vi "Main.vi"() -> ()   [LabVIEW 2021]
doc: "This vi acts as an user interface to display acquire data and save data when required. User can ineract with the panel to choose file (CSV or TDMS) and data display type(chart or graph). It also allow user to select channel index and define channel name, scale and offset. It then can let user choose a moment to start recording either on defined time length or user choice. Additional functionality of a control loop for the Cryocooler Instron project."
uses:
  Control/Data Display Choice Enum.ctl
  Control/File Choice Enum.ctl
  Control/User Interface Reference Cluster.ctl
  Control/Output Data Cluster.ctl
  Control/Command and Data Cluster.ctl
  Control/Data Display Manager Enum.ctl
  Control/Volt Chl.ctl
  Control/File Manager Enum.ctl
  Control/DAQ Manager Enum.ctl
  <vilib>/Analysis/baseanly.llb/Mean (DBL).vi
  <extravilib>/ChannelInstances/Tag-bool/Write With Abort.vi
  <extravilib>/ChannelInstances/Tag-a[.](wfm(dbl))/Read With Abort.vi
  <extravilib>/ChannelInstances/Tag-bool/Read With Abort.vi
  <extravilib>/ChannelInstances/Stream-a[.](wfm(dbl))/Read With Abort.vi
  <extravilib>/ChannelInstances/Tag-a[.](wfm(dbl))/Write With Abort.vi
  <extravilib>/ChannelInstances/Stream-a[.](wfm(dbl))/Write With Abort.vi
  <extravilib>/ChannelInstances/Stream-a[.](wfm(dbl))/EndpointRead.vi
  <extravilib>/ChannelInstances/Stream-a[.](wfm(dbl))/Endpoint.vi
  <extravilib>/ChannelInstances/Tag-bool/Instantiate.vi
  <extravilib>/ChannelInstances/Tag-a[.](wfm(dbl))/Instantiate.vi
  <extravilib>/ChannelInstances/Stream-a[.](wfm(dbl))/Instantiate.vi
  <extravilib>/ChannelInstances/Event Messenger-t'Command and Data Cluster.ctl'/Instantiate.vi
  <extravilib>/ChannelInstances/Event Messenger-t'Command and Data Cluster.ctl'/))Channel.vi
  <extravilib>/ChannelInstances/Tag-a[.](wfm(dbl))/EndpointRead.vi
  <extravilib>/ChannelInstances/Tag-bool/EndpointRead.vi
  <vilib>/Instr/_visa.llb/VISA Configure Serial Port (Instr).vi
  <vilib>/DAQmx/create/channels.llb/DAQmx Create Channel (DO-Digital Output).vi
  <extravilib>/ChannelInstances/Stream-a[.](wfm(dbl))/)Channel.vi
  <resource>/ChannelSupport/_ChannelSupport/WaitIfNeeded.vi
  <extravilib>/ChannelInstances/Tag-a[.](wfm(dbl))/Endpoint.vi
  <extravilib>/ChannelInstances/Tag-bool/Endpoint.vi
  <extravilib>/ChannelInstances/Event Messenger-t'Command and Data Cluster.ctl'.lvlib
  <extravilib>/ChannelInstances/Stream-a[.](wfm(dbl)).lvlib
  <vilib>/Analysis/NI_AALBase.lvlib
  <extravilib>/ChannelInstances/Tag-a[.](wfm(dbl)).lvlib
  <extravilib>/ChannelInstances/Tag-bool.lvlib
  <resource>/objmgr/daqmx.rc
panel:
  out "mean":dbl format="%0.2f"
  out "First read tag":waveform(dbl)[](array[waveform])
  out "not increment":bool
  out "Increment":bool
  out ".not. x?":bool
  in  "Delta T":dbl
  out "n":dbl
  out "In End?":bool
  out "Waveform Chart 2":dbl[](graph)
  out "T0":dbl
  out "T Chl 0":dbl
  out "T Chl 7":dbl
  out "Total Range 2":dbl
  in  "Lines":tag
  in  "COM Port":refnum<visa-resource-name>
  in  "Total Range":dbl
  out "Error":errorcluster
  out "Overall Raw \nVoltage Mean":dbl[](array[numeric])
  out "Raw Voltage Mean \nper Second":dbl[](array[numeric])
  out "Recording":bool
  in  "File Choice":T1
  in  "DD Choice":T2 caption="Data Display Choice"
  out "File Path":path
  in  "Choice Ok":bool
  in  "File Name":string
  in  "Exit":bool
  in  "Use Re Time":bool caption="Use Record Time"
  in  "Re Time":dbl=10.0 caption="Record Time (s)"
  in  "Device Name":tag
  in  "Sample Rate":i32=100 caption="Sample Rate (S/s)"
  in  "Init Button":bool
  in  "Record":bool
  in  "Start":bool
  in  "Stop":bool
  out "element":waveform(dbl)[](array[waveform])
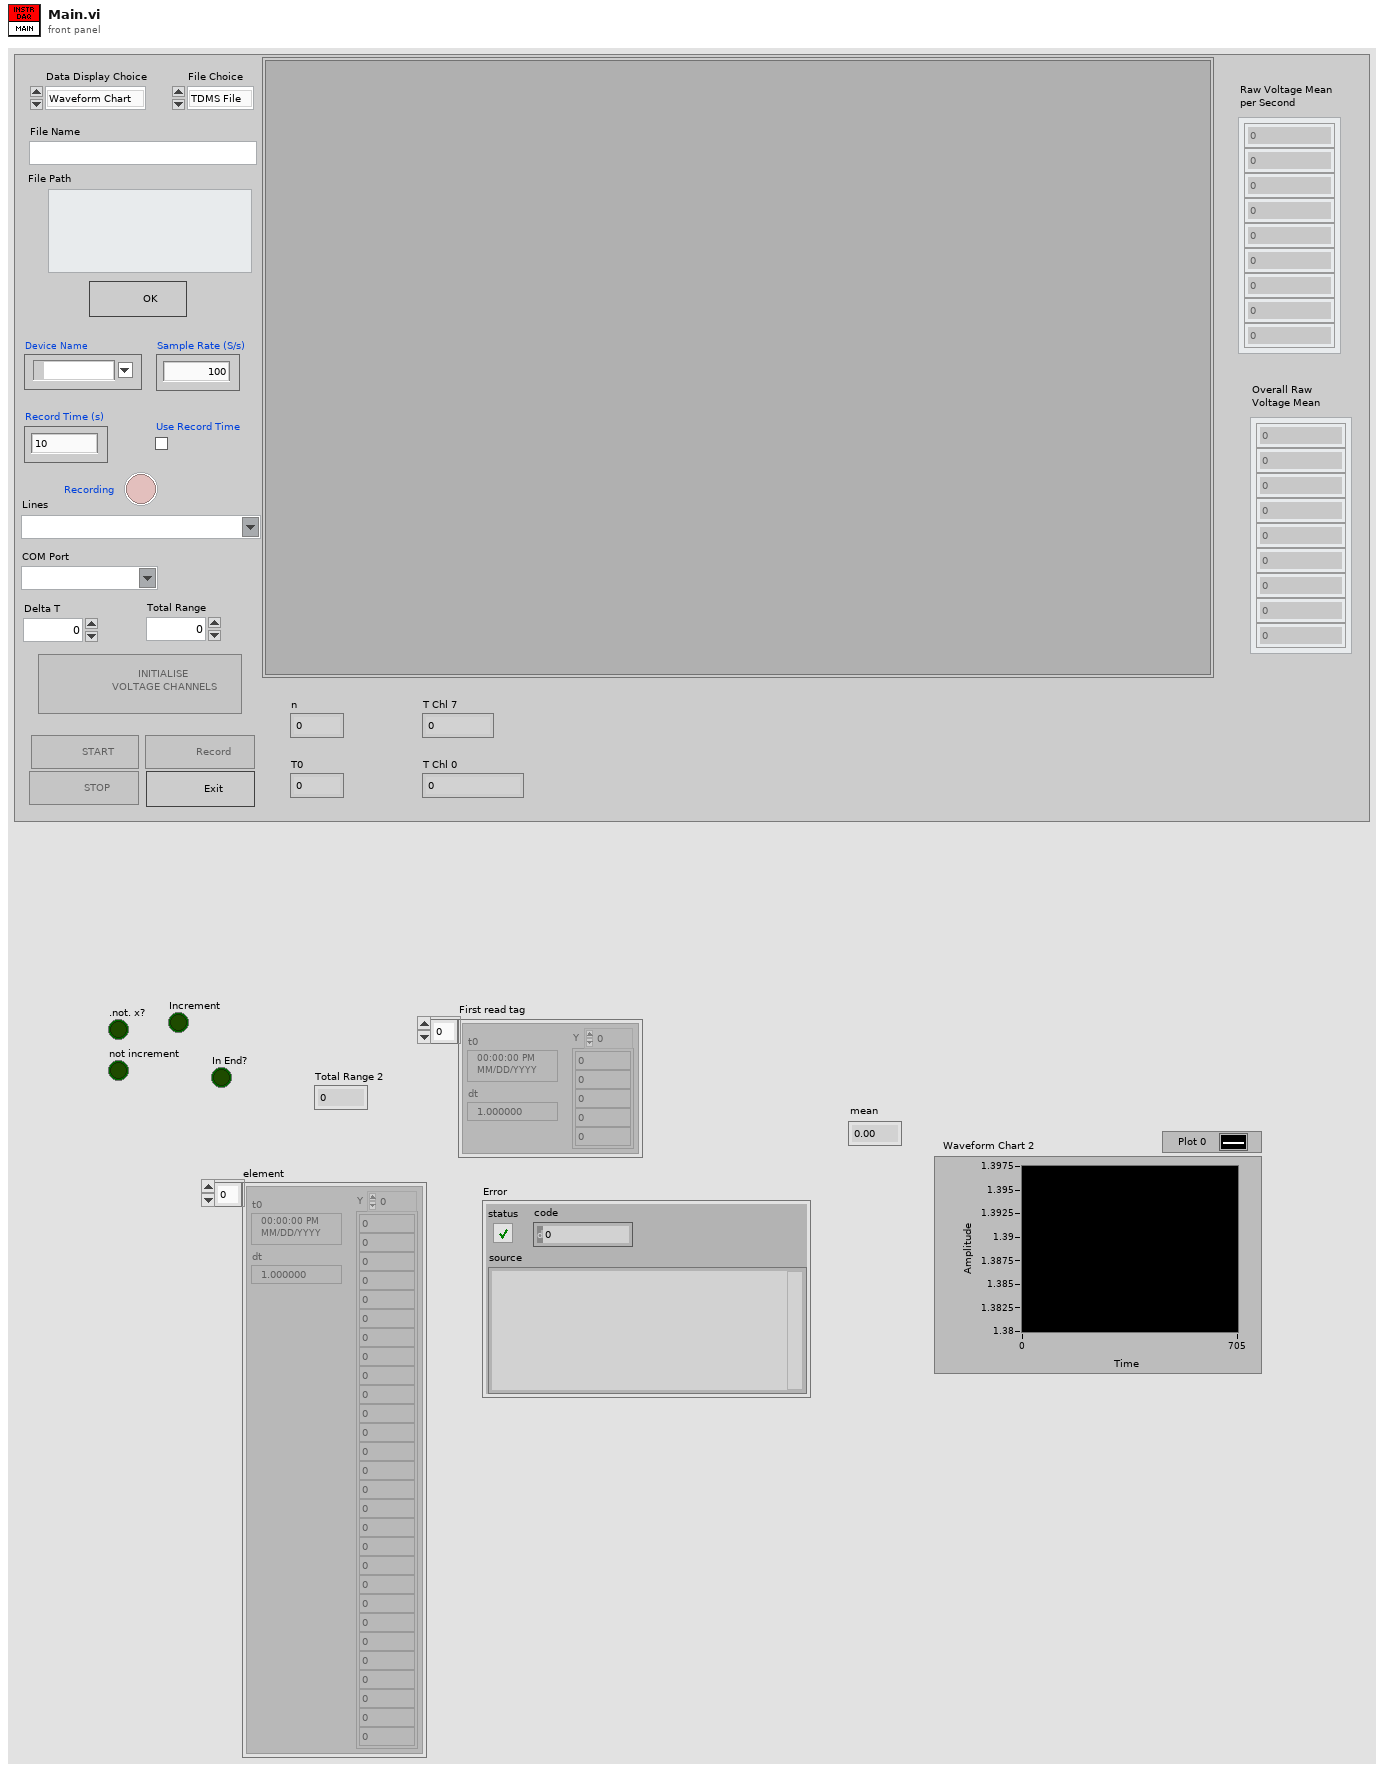
[diagram p1: front panel]
types:
  T1 = typedef "File Choice Enum.ctl" = enum16{"TDMS File", "CSV File"}
  T2 = typedef "Data Display Choice Enum.ctl" = enum16{"Waveform Chart", "Waveform Graph"}
  T3 = typedef "Command and Data Cluster.ctl" = cluster{"Command":string, "Data":variant, "Data 2":variant, "Data 3":variant, "Data 4":variant}
  T4 = typedef "Output Data Cluster.ctl" = cluster{"Digital":cluster{"DAQmx Task":refnum<k21>}, "Serial":cluster{"VISA name":refnum<visa-resource-name>}, "Total Range":dbl}
  T5 = typedef "User Interface Reference Cluster.ctl" = cluster{"Choice Ok":refnum<vi>, "Init Button":refnum<vi>, "Start":refnum<vi>, "Record":refnum<vi>, "Stop":refnum<vi>, "Exit":refnum<vi>, "File Choice":refnum<vi>, "DD Choice":refnum<vi>}
  T6 = typedef "Event Messenger-t'Command and Data Cluster.ctl'.lvlib/))Channel.ctl" = refnum<queue>
  T7 = typedef "Tag-bool.lvlib/))Channel.ctl" = refnum<queue>
  T8 = typedef "DAQ Manager Enum.ctl" = enum16{"Config", "Start", "Read", "Stop"}
  T9 = typedef "Volt Chl.ctl" = cluster{"Index":i32[], "Chl Name":string[], "Scale":dbl[], "Offset":dbl[], "Sample Rate":i32, "Device Name":tag, "Channel":tag}
  T10 = typedef "Stream-a[.](wfm(dbl)).lvlib/)Channel.ctl" = refnum<queue>
  T11 = typedef "Tag-a[.](wfm(dbl)).lvlib/))Channel.ctl" = refnum<queue>
  T12 = typedef "File Manager Enum.ctl" = enum16{"Create File", "Config Data", "Volt Data", "Close File"}
  T13 = typedef "Data Display Manager Enum.ctl" = enum16{"Display Choice", "Config Data", "Volt Data"}
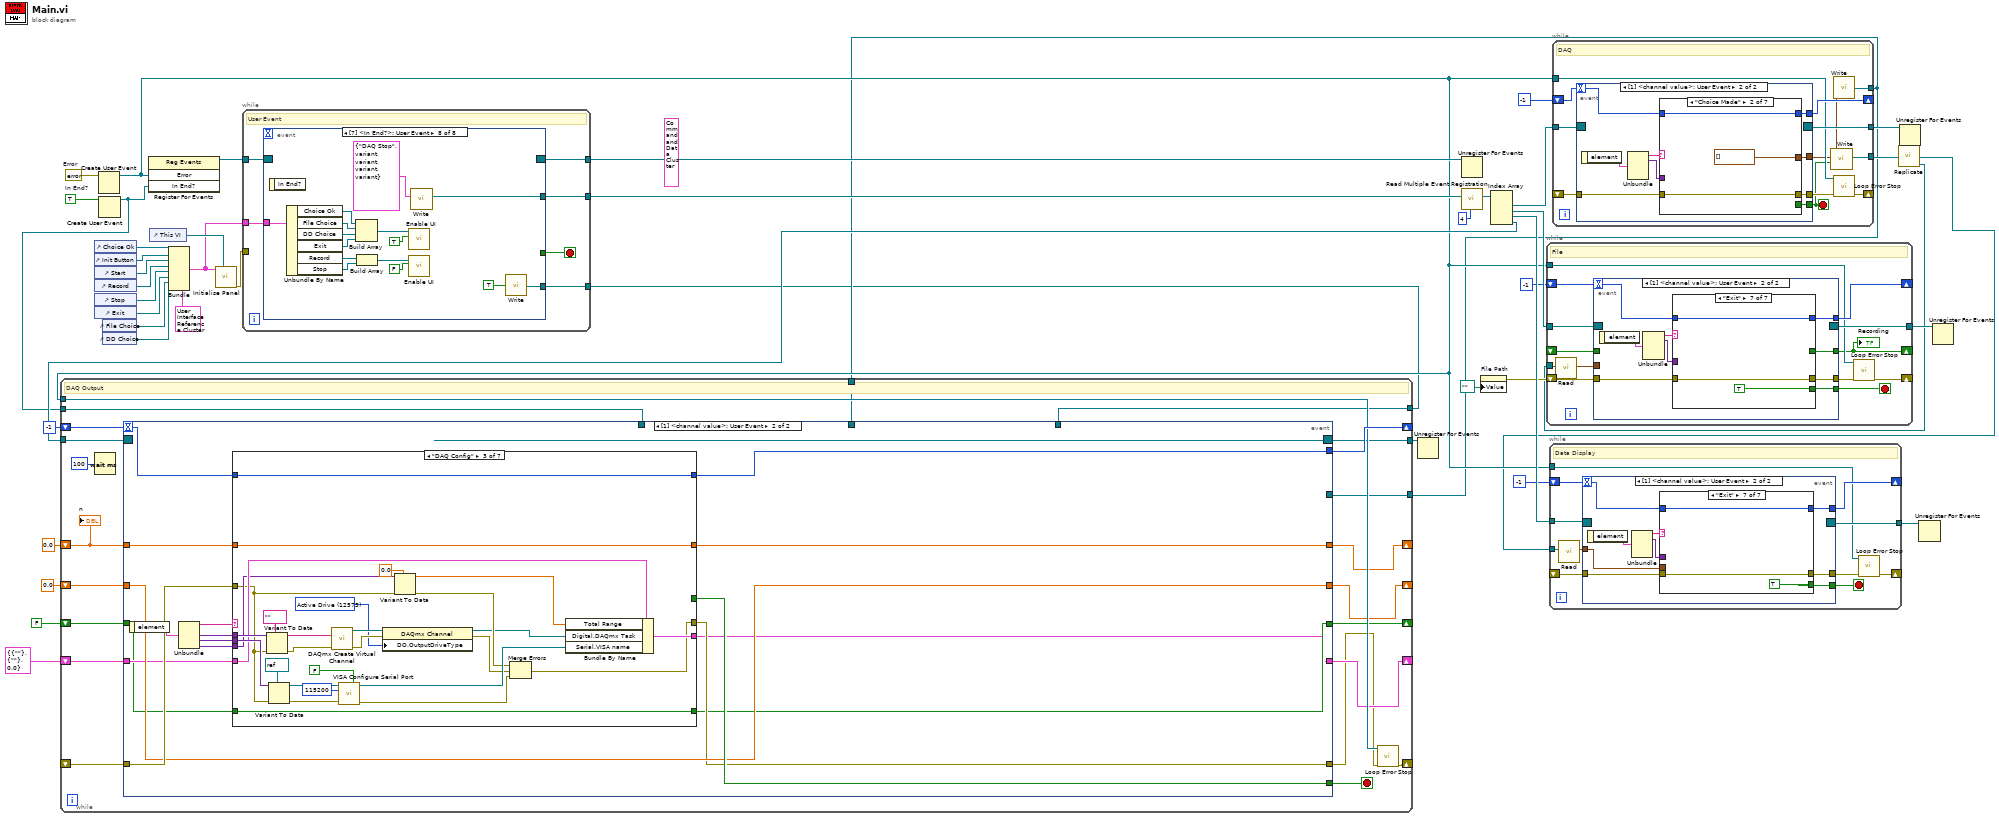
[diagram p0: block diagram]
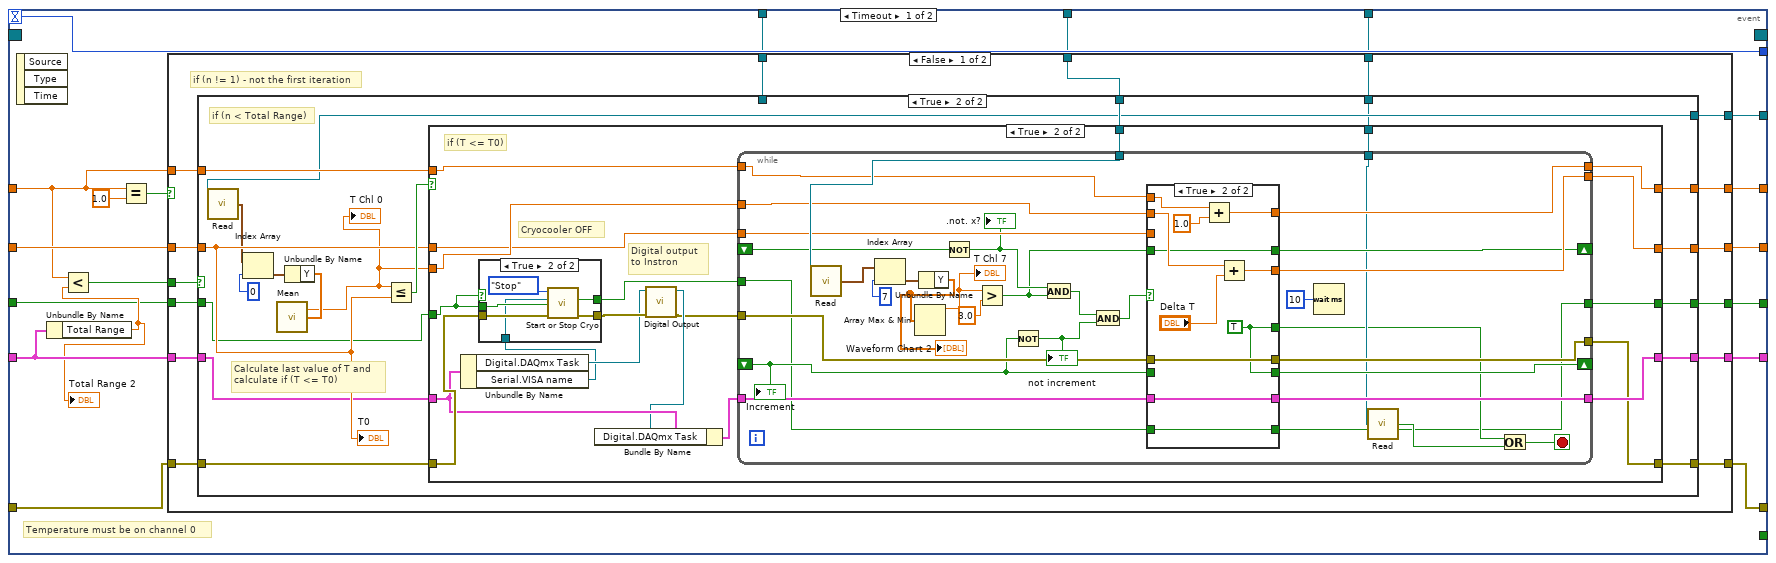
[diagram p2: hidden frame]
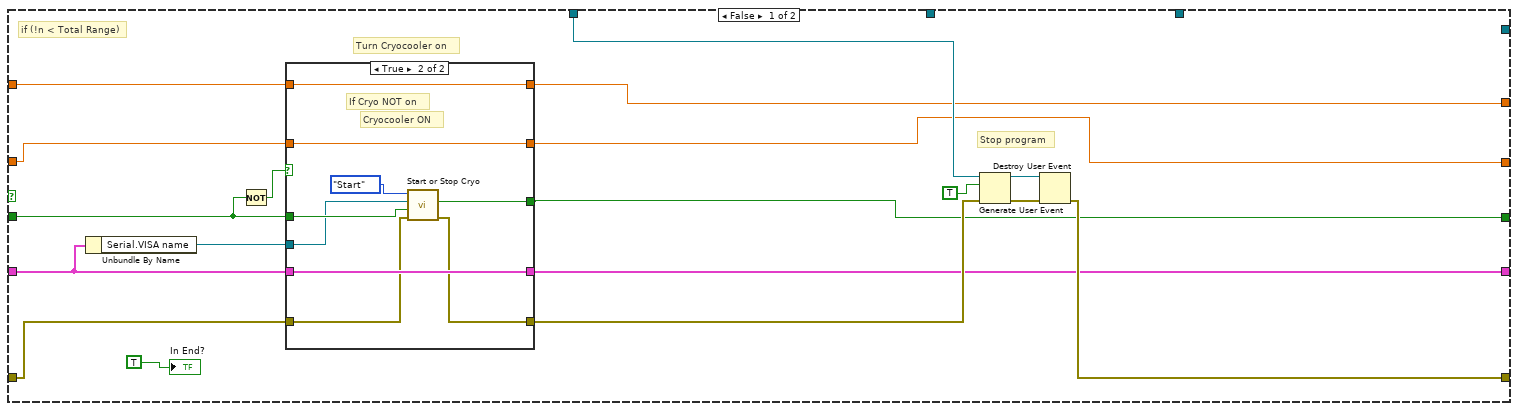
[diagram p3: hidden frame]
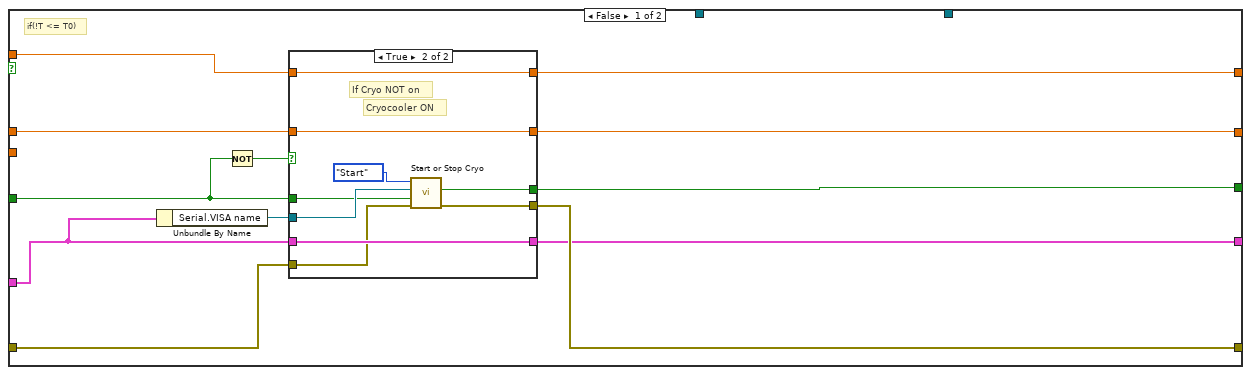
[diagram p5: hidden frame]
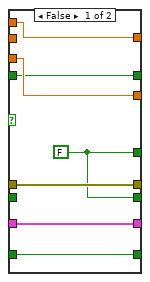
[diagram p8: hidden frame]
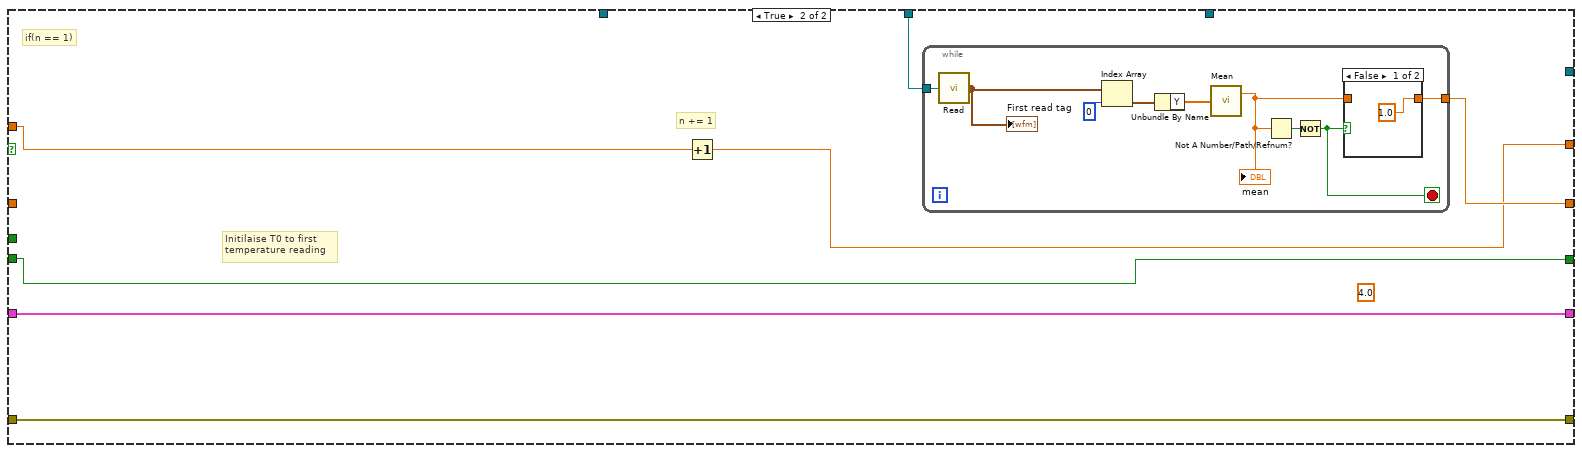
[diagram p9: hidden frame]
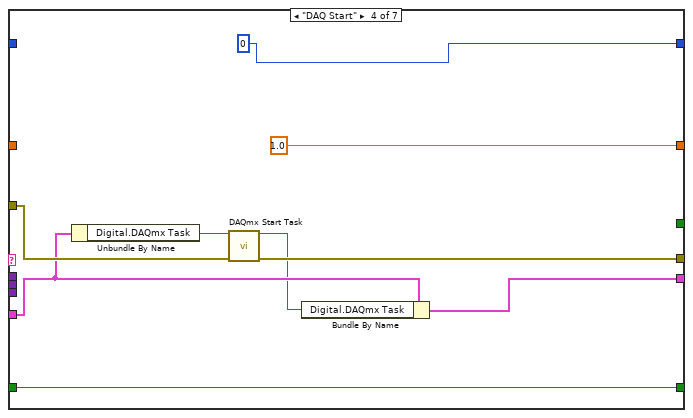
[diagram p13: hidden frame]
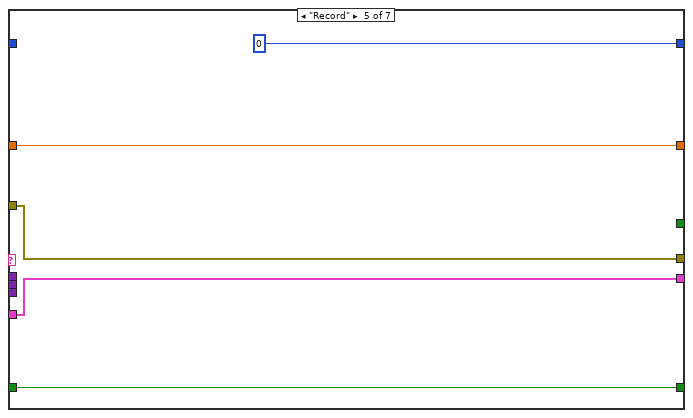
[diagram p14: hidden frame]
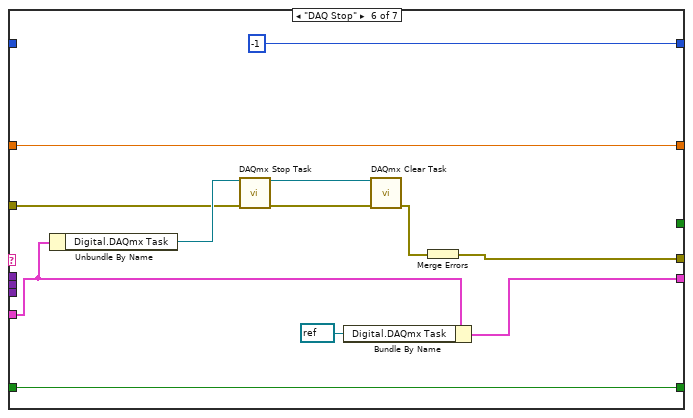
[diagram p15: hidden frame]
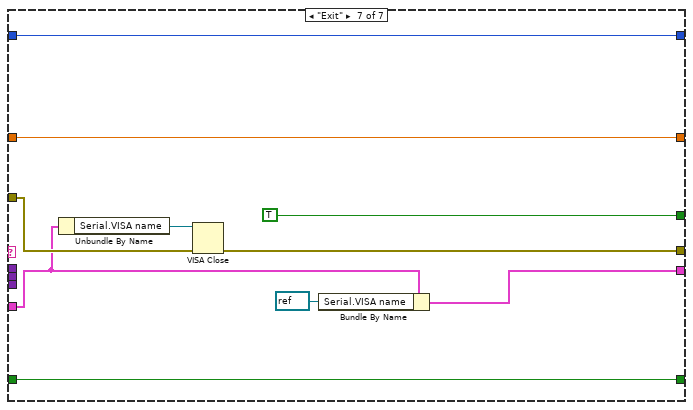
[diagram p16: hidden frame]
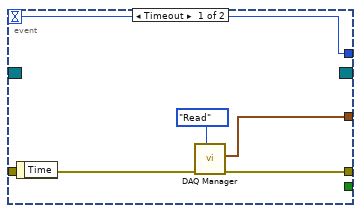
[diagram p17: hidden frame]
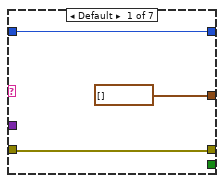
[diagram p18: hidden frame]
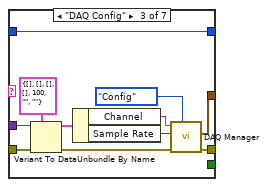
[diagram p19: hidden frame]
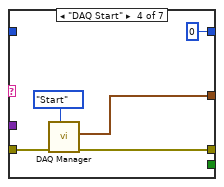
[diagram p20: hidden frame]
diagram:
  w2 = TRUE  # In End?
  (unwired) T3 {"Command"="DAQ Stop", "Data"=variant, "Data 2"=variant, "Data 3"=variant, "Data 4"=variant} ("Cluster")
  w16 = errorcluster {"status"=FALSE, "code"=0, "source"=""}  # Error
  n1 = control-ref of="Choice Ok"() -> (w31:refnum<vi>)
  n2 = control-ref of="Init Button"() -> (w30:refnum<vi>)
  n3 = control-ref of="Start"() -> (w29:refnum<vi>)
  n4 = control-ref of="Record"() -> (w28:refnum<vi>)
  n5 = control-ref of="Stop"() -> (w27:refnum<vi>)
  n6 = control-ref of="Exit"() -> (w26:refnum<vi>)
  n7 = Create User Event(user event datatype=w16) -> (user event=w13:refnum<user-event>)  [unwired: 1 in, 1 out]
  n8 = Create User Event(user event datatype=w2) -> (user event=w1:refnum<user-event>)  [unwired: 1 in, 1 out]
  n9 = control-ref of="File Choice"() -> (w25:refnum<vi>)
  n10 = control-ref of="DD Choice"() -> (w24:refnum<vi>)
  n11 = register-events(w13, w1) -> (reference out=w19:refnum<event-registration>)  [unwired: 2 in, 1 out]
  n12 = control-ref of="This VI"() -> (w17:refnum<vi>)
  n13 = Bundle(cluster=T5 {"Choice Ok"=refnum, "Init Button"=refnum, "Start"=refnum, "Record"=refnum, "Stop"=refnum, "Exit"=refnum, "File Choice"=refnum, "DD Choice"=refnum} ("output cluster"), "Choice Ok"=w31, "Init Button"=w30, "Start"=w29, "Record"=w28, "Stop"=w27, "Exit"=w26, "File Choice"=w25, "DD Choice"=w24) -> (w3:T5)
  n14 = call "Initialise Panel.vi"("This VI"=w17, "UI Ref"=w3) -> ("error out"=w22:errorcluster)  [unwired: 9 in]
  n15 = while {
    tunnel: [w49] -> w38
    tunnel: w22 -> [_]
    tunnel: w3 -> [w48]
    tunnel: w19 -> [w47]
    tunnel: [w46] -> w18
    tunnel: [w45] -> w5
    stop <- w50 stop-if-true
    # "User Event"
    n16 = event shown="[7] <In End?>: User Event" {
      selector: w47 -> [_ _ _ _ _ _ _ _]
      dyn-events: [_ _ _ _ _ _ _ _] -> w46
      timeout: _ -> [_ _ _ _ _ _ _ _]
      tunnel: [TRUE TRUE _ _ _ _ _ _] -> w50
      tunnel: [w51 w59 w71 w90 w103 w109 w123 w138] -> w49
      tunnel: w48 -> [_ _ w70 w85 w95 w104 w122 w137]
      tunnel: [_ _ _ _ _ _ w110 w125] -> w45
      event "Exit": Value Change {
        n17 = event-data() -> ()  [unwired: 1 in, 1 out]
        n18 = call <extravilib>:"Write.vi"("element"=T3 {"Command"="Exit", "Data"=variant, "Data 2"=variant, "Data 3"=variant, "Data 4"=variant} ("Cluster")) -> ("channel"=w51:T6)  [unwired: 9 in, 1 out]
      }
      event User Event {
        w58 = errorcluster {"status"=FALSE, "code"=0, "source"=""}  # Error
        n19 = event-data() -> ("status"=w57:bool, "code"=w56:i32, "source"=w55:string)  [unwired: 1 in]
        n20 = Bundle(cluster=w58, "status"=w57, "code"=w56, "source"=w55) -> (→"Error":errorcluster)
        n21 = call <extravilib>:"Write.vi"("element"=T3 {"Command"="Exit", "Data"=variant, "Data 2"=variant, "Data 3"=variant, "Data 4"=variant} ("Cluster")) -> ("channel"=w59:T6)  [unwired: 9 in, 1 out]
      }
      event "Choice Ok": Value Change {
        n22 = event-data() -> ()  [unwired: 1 in, 1 out]
        n23 = Unbundle By Name(w70) -> ("File Choice"=w63:refnum<vi>, "DD Choice"=w62:refnum<vi>, "Choice Ok"=w69:refnum<vi>, "Init Button"=w68:refnum<vi>)
        n24 = Build Array(w63, w62, w69) -> (w66:refnum<vi>[])
        n25 = Build Array(w68) -> (w64:refnum<vi>[])
        n26 = call <extravilib>:"Write.vi"("element"=T3 {"Command"="Choice Made", "Data"=variant, "Data 2"=variant, "Data 3"=variant, "Data 4"=variant} ("Cluster")) -> ("channel"=w71:T6)  [unwired: 9 in, 1 out]
        n27 = call "Enable UI.vi"("Enable?"=FALSE, "output cluster"=w66) -> ()  [unwired: 9 in, 1 out]
        n28 = call "Enable UI.vi"("Enable?"=TRUE, "output cluster"=w64) -> ()  [unwired: 9 in, 1 out]
      }
      event "Init Button": Value Change {
        n29 = event-data() -> ()  [unwired: 1 in, 1 out]
        n30 = Unbundle By Name(w85) -> ("Init Button"=w80:refnum<vi>, "Start"=w79:refnum<vi>)
        n31 = Build Array(w79) -> (w83:refnum<vi>[])
        n32 = Build Array(w80) -> (w84:refnum<vi>[])
        n33 = To Variant(anything="COM Port") -> (Variant=w77:variant)
        n34 = To Variant(anything="Lines") -> (Variant=w75:variant)
        n35 = call "DAQ Channel Dlg_V0.vi"("DAQ Sample Rate (S/s)"="Sample Rate", "Device Name"="Device Name") -> ("Chl Infor"=w86:variant)  [unwired: 9 in]
        n36 = call "Enable UI.vi"("Enable?"=FALSE, "output cluster"=w84) -> ()  [unwired: 9 in, 1 out]
        n37 = call "Enable UI.vi"("Enable?"=TRUE, "output cluster"=w83) -> ()  [unwired: 9 in, 1 out]
        n38 = To Variant(anything="Total Range") -> (Variant=w73:variant)
        n39 = Bundle(cluster=T3 {"Command"="DAQ Config", "Data"=variant, "Data 2"=variant, "Data 3"=variant, "Data 4"=variant} ("Cluster"), "Command"="DAQ Config" ("element"), "Data"=w86, "Data 2"=w75, "Data 3"=w77, "Data 4"=w73) -> (w88:T3)
        n40 = call <extravilib>:"Write.vi"("element"=w88) -> ("channel"=w90:T6)  [unwired: 9 in, 1 out]
      }
      event "Start": Value Change {
        n41 = event-data() -> ()  [unwired: 1 in, 1 out]
        n42 = Unbundle By Name(w95) -> ("Exit"=w93:refnum<vi>, "Start"=w97:refnum<vi>, "Record"=w96:refnum<vi>, "Stop"=w94:refnum<vi>)
        n43 = Build Array(w93, w97) -> (w101:refnum<vi>[])
        n44 = Build Array(w96, w94) -> (w100:refnum<vi>[])
        n45 = call "Enable UI.vi"("Enable?"=FALSE, "output cluster"=w101) -> ()  [unwired: 9 in, 1 out]
        n46 = call "Enable UI.vi"("Enable?"=TRUE, "output cluster"=w100) -> ()  [unwired: 9 in, 1 out]
        n47 = call <extravilib>:"Write.vi"("element"=T3 {"Command"="DAQ Start", "Data"=variant, "Data 2"=variant, "Data 3"=variant, "Data 4"=variant} ("Cluster")) -> ("channel"=w103:T6)  [unwired: 9 in, 1 out]
      }
      event "Record": Value Change {
        n48 = event-data() -> ()  [unwired: 1 in, 1 out]
        n49 = Unbundle By Name(w104) -> ("Record"=w105:refnum<vi>)
        n50 = Build Array(w105) -> (w107:refnum<vi>[])
        n51 = call "Enable UI.vi"("Enable?"=FALSE, "output cluster"=w107) -> ()  [unwired: 9 in, 1 out]
        n52 = call <extravilib>:"Write.vi"("element"=T3 {"Command"="Record", "Data"=variant, "Data 2"=variant, "Data 3"=variant, "Data 4"=variant} ("Cluster")) -> ("channel"=w109:T6)  [unwired: 9 in, 1 out]
      }
      event "Stop": Value Change {
        n53 = event-data() -> ()  [unwired: 1 in, 1 out]
        n54 = Unbundle By Name(w122) -> ("Choice Ok"=w118:refnum<vi>, "File Choice"=w119:refnum<vi>, "DD Choice"=w120:refnum<vi>, "Exit"=w116:refnum<vi>, "Record"=w115:refnum<vi>, "Stop"=w112:refnum<vi>)
        n55 = Build Array(w118, w119, w120, w116) -> (w117:refnum<vi>[])
        n56 = Build Array(w115, w112) -> (w113:refnum<vi>[])
        n57 = call "Enable UI.vi"("Enable?"=TRUE, "output cluster"=w117) -> ()  [unwired: 9 in, 1 out]
        n58 = call "Enable UI.vi"("Enable?"=FALSE, "output cluster"=w113) -> ()  [unwired: 9 in, 1 out]
        n59 = call <extravilib>:"Write.vi"("element"=T3 {"Command"="DAQ Stop", "Data"=variant, "Data 2"=variant, "Data 3"=variant, "Data 4"=variant} ("Cluster")) -> ("channel"=w123:T6)  [unwired: 9 in, 1 out]
        n60 = call <extravilib>:"Write.vi"("element"=TRUE) -> ("channel"=w110:T7)  [unwired: 1 out]
      }
      event User Event {
        n61 = event-data() -> ()  [unwired: 1 in, 1 out]
        n62 = Unbundle By Name(w137) -> ("Choice Ok"=w133:refnum<vi>, "File Choice"=w134:refnum<vi>, "DD Choice"=w135:refnum<vi>, "Exit"=w131:refnum<vi>, "Record"=w130:refnum<vi>, "Stop"=w127:refnum<vi>)
        n63 = Build Array(w133, w134, w135, w131) -> (w132:refnum<vi>[])
        n64 = Build Array(w130, w127) -> (w128:refnum<vi>[])
        n65 = call "Enable UI.vi"("Enable?"=TRUE, "output cluster"=w132) -> ()  [unwired: 9 in, 1 out]
        n66 = call "Enable UI.vi"("Enable?"=FALSE, "output cluster"=w128) -> ()  [unwired: 9 in, 1 out]
        n67 = call <extravilib>:"Write.vi"("element"=T3 {"Command"="DAQ Stop", "Data"=variant, "Data 2"=variant, "Data 3"=variant, "Data 4"=variant} ("Cluster")) -> ("channel"=w138:T6)  [unwired: 9 in, 1 out]
        n68 = call <extravilib>:"Write.vi"("element"=TRUE) -> ("channel"=w125:T7)  [unwired: 1 out]
      }
    }
  }
  n69 = Unregister For Events(event registration refnum=w18) -> ()  [unwired: 1 in, 1 out]
  n70 = call <extravilib>:"Read Multiple Event Registration.vi"("number of event structures"=u16 4, "channel"=w38) -> ("event registration refnums"=w36:refnum<event-registration>[])  [unwired: 9 in]
  n71 = property on="File Path" class="Path"("Value"=path "" ("File Path")) -> (error out=w20:errorcluster)  [unwired: 2 in, 1 out]
  n72 = Index Array(array=w36) -> (element #1=w42:refnum<event-registration>, element #2=w43:refnum<event-registration>, element #3=w41:refnum<event-registration>, element #4=w15:refnum<event-registration>)  [unwired: 4 in]
  n73 = while {
    tunnel: w42 -> [w151]
    tunnel: [w150] -> w39
    shift-right: [w148] -> _
    shift-left: -1 -> [w149]
    tunnel: [w143] -> w33
    shift-right: [w145] -> _
    shift-left: _ -> [w147]
    tunnel: w13 -> [w146]
    tunnel: [w140] -> w6
    stop <- w141 stop-if-true
    # "DAQ"
    n74 = event shown="[1] <channel value>: User Event" {
      selector: w151 -> [_ _]
      dyn-events: [_ _] -> w150
      timeout: w149 -> [w156 w160]
      tunnel: [w155 w165] -> w144
      tunnel: [_ w164] -> w141
      tunnel: [w156 w159] -> w148
      tunnel: w147 -> [w153 w158]
      tunnel: [w152 w157] -> w142
      event Timeout {
        n75 = event-data() -> ()  [unwired: 1 in, 1 out]
        n76 = call "DAQ Manager.vi"("Enum"=DAQ_Manager_Enum."Read", "error in"=w153) -> ("error out"=w155:errorcluster, "data"=w152:waveform(dbl)[])  [unwired: 8 in]
      }
      event User Event {
        n77 = event-data() -> ("element"=w163:T3)  [unwired: 1 in]
        n78 = Unbundle(w163) -> ("Command"=w162:string, "Data"=w161:variant)  [unwired: 3 out]
        n79 = case shown="\"Choice Made\"" w162 {
          tunnel: [w167 w170 w175 w186 w188 w195 w199] -> w165
          tunnel: [_ _ _ _ _ _ TRUE] -> w164
          tunnel: w161 -> [_ _ w182 _ _ _ _]
          tunnel: w160 -> [w168 w171 w174 _ _ _ w201]
          tunnel: [w168 w171 w174 0 0 -1 w201] -> w159
          tunnel: w158 -> [w167 w170 w173 w184 w189 w194 w199]
          tunnel: [waveform(dbl)[] [] ("element") waveform(dbl)[] [] ("element") w172 w183 w190 w193 waveform(dbl)[] [] ("element")] -> w157
          frame Default {
          }
          frame "Choice Made" {
          }
          frame "DAQ Config" {
            n80 = Variant To Data(error in=w173, type=T9 {"Index"=[], "Chl Name"=[], "Scale"=[], "Offset"=[], "Sample Rate"=100, "Device Name"="", "Channel"=""} ("Volt Channel"), Variant=w182) -> (data=w180:T9, error out=w177:errorcluster)
            n81 = Unbundle By Name(w180) -> ("Channel"=w179:tag, "Sample Rate"=w178:i32)
            n82 = call "DAQ Manager.vi"("Enum"=DAQ_Manager_Enum."Config", "error in"=w177, "Sample Rate"=w178, "Chl"=w179) -> ("error out"=w175:errorcluster, "data"=w172:waveform(dbl)[])  [unwired: 6 in]
          }
          frame "DAQ Start" {
            n83 = call "DAQ Manager.vi"("Enum"=DAQ_Manager_Enum."Start", "error in"=w184) -> ("error out"=w186:errorcluster, "data"=w183:waveform(dbl)[])  [unwired: 8 in]
          }
          frame "Record" {
            n84 = call "DAQ Manager.vi"("Enum"=DAQ_Manager_Enum."Read", "error in"=w189) -> ("error out"=w188:errorcluster, "data"=w190:waveform(dbl)[])  [unwired: 8 in]
          }
          frame "DAQ Stop" {
            n85 = call "DAQ Manager.vi"("Enum"=DAQ_Manager_Enum."Stop", "error in"=w194) -> ("error out"=w195:errorcluster, "data"=w193:waveform(dbl)[])  [unwired: 8 in]
          }
          frame "Exit" {
          }
        }
      }
    }
    n86 = call <extravilib>:"Write.vi"("last element? (F)"=w141, "element"=w142) -> ("channel"=w143:T10)  [unwired: 7 in, 2 out]
    n87 = call <extravilib>:"Write.vi"("element"=w142) -> ("channel"=w140:T11)  [unwired: 1 out]
    n88 = call "Loop Error Stop.vi"("error in"=w144, "user event"=w146) -> ("error out"=w145:errorcluster)  [unwired: 9 in]
  }
  n89 = while {
    tunnel: w15 -> [w223]
    shift-right: [w221] -> _
    shift-left: -1 -> [w222]
    shift-right: [w220] -> _
    shift-left: _ -> [w219]
    tunnel: w13 -> [w218]
    tunnel: [w217] -> w12
    shift-right: [w209] -> _
    shift-left: 0.0 -> [w215]
    shift-right: [w208] -> _
    shift-left: 0.0 -> [w214]
    shift-right: [w211] -> _
    shift-left: T4 {"Digital"={"DAQmx Task"=""}, "Serial"={"VISA name"=""}, "Total Range"=0.0} ("Output Data") -> [w213]
    tunnel: w6 -> [w212]
    tunnel: w6 -> [w206]
    tunnel: w5 -> [w205]
    shift-right: [w203] -> _
    shift-left: FALSE -> [w204]
    tunnel: w1 -> [w202]
    stop <- w216 stop-if-true
    # "DAQ Output"
    n90 = Wait (ms)(milliseconds to wait=u32 100) -> ()  [unwired: 1 out]
    n91 = event shown="[1] <channel value>: User Event" {
      selector: w223 -> [_ _]
      dyn-events: [_ _] -> w217
      timeout: w222 -> [w242 w445]
      tunnel: [w242 w444] -> w221
      tunnel: w219 -> [w233 w443]
      tunnel: [_ w442] -> w216
      tunnel: w215 -> [w235 w440]
      tunnel: w214 -> [w237 w439]
      tunnel: [w236 w441] -> w209
      tunnel: [w239 w439] -> w208
      tunnel: w213 -> [w232 w436]
      tunnel: [w234 w431] -> w211
      tunnel: [w229 w435] -> w207
      tunnel: w212 -> [w230 _]
      tunnel: w206 -> [w228 _]
      tunnel: w205 -> [w227 _]
      tunnel: w204 -> [w226 w433]
      tunnel: [w225 w432] -> w203
      tunnel: w202 -> [w224 _]
      event Timeout {
        # "Temperature must be on channel 0"
        n92 = event-data() -> ()  [unwired: 1 in, 3 out]
        n93 = Unbundle By Name(w232) -> ("Total Range"=w231:dbl)
        "Total Range 2" <- w231
        n94 = Less?(x=w235, y=w231) -> (x < y?=w238:bool)
        n95 = Equal?(x=w235, y=1.0) -> (x = y?=w240:bool)
        n96 = case shown="False" w240 {
          tunnel: [w255 w415] -> w239
          tunnel: w238 -> [w257 _]
          tunnel: w237 -> [w256 _]
          tunnel: [w254 w414] -> w236
          tunnel: w235 -> [w253 w417]
          tunnel: w232 -> [w252 w419]
          tunnel: [w251 w419] -> w234
          tunnel: w233 -> [w250 w418]
          tunnel: [w249 w418] -> w229
          tunnel: w230 -> [w248 w416]
          tunnel: w228 -> [w247 _]
          tunnel: w227 -> [w246 _]
          tunnel: w226 -> [w245 w413]
          tunnel: [w244 w413] -> w225
          tunnel: w224 -> [w243 _]
          frame False {
            # "if (n != 1) - not the first iteration"
            n97 = case shown="True" w257 {
              tunnel: w256 -> [w267 w302]
              tunnel: [w266 w305] -> w255
              tunnel: [w268 w304] -> w254
              tunnel: w253 -> [w269 w303]
              tunnel: w252 -> [w259 w301]
              tunnel: [w262 w300] -> w251
              tunnel: w250 -> [w265 w299]
              tunnel: [w270 w298] -> w249
              tunnel: w248 -> [_ w295]
              tunnel: w247 -> [_ w294]
              tunnel: w246 -> [_ w292]
              tunnel: w245 -> [w261 w291]
              tunnel: [w263 w290] -> w244
              tunnel: w243 -> [w274 _]
              frame False {
                # "Turn Cryocooler on"
                # "Stop program"
                # "if (!n < Total Range)"
                n98 = Unbundle By Name(w259) -> ("Serial.VISA name"=w258:refnum<visa-resource-name>)
                n99 = Not(x=w261) -> (.not. x?=w260:bool)
                n100 = case shown="True" w260 {
                  tunnel: [w280 w288] -> w263
                  tunnel: w269 -> [w277 w287]
                  tunnel: [w277 w287] -> w268
                  tunnel: w267 -> [w276 w286]
                  tunnel: [w276 w286] -> w266
                  tunnel: w261 -> [w280 w284]
                  tunnel: w259 -> [w279 w285]
                  tunnel: [w279 w285] -> w262
                  tunnel: w265 -> [w278 w282]
                  tunnel: [w278 w281] -> w264
                  tunnel: w258 -> [_ w283]
                  frame False {
                  }
                  frame True {
                    # "If Cryo NOT on"
                    # "Cryocooler ON"
                    n101 = call "Start or Stop Cryo.vi"("error in"=w282, "On?"=w284, "VISA resource name"=w283, "State"=enum16{"Start", "Stop"}."Start") -> ("error out"=w281:errorcluster, "On? Out"=w288:bool)  [unwired: 5 in, 1 out]
                  }
                }
                n102 = Generate User Event(user event=w274, event data cluster=TRUE ("event data"), error in=w264) -> (user event out=w273:refnum<user-event>, error out=w271:errorcluster)  [unwired: 1 in]
                n103 = Destroy User Event(user event=w273, error in=w271) -> (error out=w270:errorcluster)
                "In End?" <- TRUE ("In End?")
              }
              frame True {
                # "Calculate last value of T and \ncalculate if (T <= T0)"
                # "if (n < Total Range)"
                n104 = call <extravilib>:"Read.vi"("channel"=w294) -> ("element"=w293:waveform(dbl)[])  [unwired: 1 in, 1 out]
                n105 = Index Array(array=w293, index=0) -> (element=w307:waveform(dbl))
                n106 = Unbundle By Name(w307) -> ("Y"=w297:dbl[])
                n107 = call-poly <vilib>:"Mean.vi"("X"=w297) -> ("mean"=w296:dbl)  [unwired: 1 out]
                "T Chl 0" <- w296
                n108 = Less Or Equal?(x=w296, y=w302) -> (x <= y?=w306:bool)
                n109 = case shown="True" w306 {
                  tunnel: [w313 w343] -> w305
                  tunnel: [w315 w344] -> w304
                  tunnel: w303 -> [w316 w354]
                  tunnel: w302 -> [w314 w340]
                  tunnel: w301 -> [w312 w350]
                  tunnel: [w311 w345] -> w300
                  tunnel: w299 -> [w319 w353]
                  tunnel: [w318 w341] -> w298
                  tunnel: w296 -> [_ w347]
                  tunnel: w295 -> [_ w346]
                  tunnel: w292 -> [_ w339]
                  tunnel: w291 -> [w310 w336]
                  tunnel: [w317 w337] -> w290
                  frame False {
                    # "if(!T <= T0)"
                    n110 = Unbundle By Name(w312) -> ("Serial.VISA name"=w320:refnum<visa-resource-name>)
                    n111 = Not(x=w310) -> (.not. x?=w309:bool)
                    n112 = case shown="True" w309 {
                      tunnel: w320 -> [_ w333]
                      tunnel: w319 -> [w322 w326]
                      tunnel: [w322 w332] -> w318
                      tunnel: w310 -> [w321 w331]
                      tunnel: [w321 w330] -> w317
                      tunnel: w316 -> [w325 w329]
                      tunnel: [w325 w329] -> w315
                      tunnel: w314 -> [w324 w328]
                      tunnel: [w324 w328] -> w313
                      tunnel: w312 -> [w323 w327]
                      tunnel: [w323 w327] -> w311
                      frame False {
                      }
                      frame True {
                        # "If Cryo NOT on"
                        # "Cryocooler ON"
                        n113 = call "Start or Stop Cryo.vi"("error in"=w326, "On?"=w331, "VISA resource name"=w333, "State"=enum16{"Start", "Stop"}."Start") -> ("error out"=w332:errorcluster, "On? Out"=w330:bool)  [unwired: 5 in, 1 out]
                      }
                    }
                  }
                  frame True {
                    # "Digital output \nto Instron"
                    # "Cryocooler OFF"
                    # "if (T <= T0)"
                    n114 = Unbundle By Name(w350) -> ("Digital.DAQmx Task"=w351:refnum<k21>, "Serial.VISA name"=w335:refnum<visa-resource-name>)
                    n115 = case shown="True" w336 {
                      tunnel: w353 -> [w356 w362]
                      tunnel: [w356 w361] -> w352
                      tunnel: w336 -> [w355 w360]
                      tunnel: [w355 w359] -> w338
                      tunnel: w335 -> [_ w357]
                      frame False {
                      }
                      frame True {
                        n116 = call "Start or Stop Cryo.vi"("error in"=w362, "On?"=w360, "VISA resource name"=w357, "State"=enum16{"Start", "Stop"}."Stop") -> ("error out"=w361:errorcluster, "On? Out"=w359:bool)  [unwired: 5 in, 1 out]
                      }
                    }
                    n117 = call "Digital Output.vi"("error in"=w352, "DAQmx Task Name"=w351) -> ("error out"=w342:errorcluster, "DAQmx Task Name Out"=w348:refnum<k21>)  [unwired: 8 in]
                    n118 = Bundle By Name(cluster=w350, "Digital.DAQmx Task"=w348) -> (w349:T4)
                    n119 = while {
                      tunnel: w347 -> [w390]
                      tunnel: w349 -> [w385]
                      tunnel: [w384] -> w345
                      tunnel: w346 -> [w394]
                      tunnel: [w389] -> w343
                      tunnel: w342 -> [w393]
                      tunnel: [w392] -> w341
                      tunnel: w340 -> [w388]
                      tunnel: w354 -> [w381]
                      tunnel: [w391] -> w344
                      shift-right: [w386] -> _
                      shift-left: _ -> [w387]
                      shift-right: [w383] -> _
                      shift-left: _ -> [w382]
                      tunnel: w339 -> [w368]
                      tunnel: w338 -> [w364]
                      tunnel: [w363] -> w337
                      stop <- w365 stop-if-true
                      n120 = call <extravilib>:"Read.vi"("channel"=w394) -> ("element"=w376:waveform(dbl)[])  [unwired: 1 in, 1 out]
                      n121 = Index Array(array=w376, index=7) -> (element=w379:waveform(dbl))
                      n122 = Unbundle By Name(w379) -> ("Y"=w375:dbl[])
                      "Waveform Chart 2" <- w375
                      n123 = Array Max & Min(array=w375) -> (max value=w377:dbl)  [unwired: 3 out]
                      "T Chl 7" <- w377
                      n124 = Not(x=w387) -> (.not. x?=w374:bool)
                      ".not. x?" <- w374
                      n125 = Greater?(x=w377, y=3.0) -> (0:w373:bool)
                      n126 = Not(x=w382) -> (.not. x?=w371:bool)
                      "not increment" <- w371
                      n127 = And(x=w374, y=w373) -> (x .and. y?=w372:bool)
                      n128 = And(x=w372, y=w371) -> (x .and. y?=w370:bool)
                      n129 = case shown="True" w370 {
                        tunnel: [w397 w408] -> w391
                        tunnel: [w401 w412] -> w392
                        tunnel: w393 -> [w401 w412]
                        tunnel: w390 -> [_ w411]
                        tunnel: [w400 w410] -> w389
                        tunnel: w388 -> [w400 _]
                        tunnel: [w396 w404] -> w366
                        tunnel: w373 -> [w399 w406]
                        tunnel: [w399 w406] -> w386
                        tunnel: w385 -> [w398 w405]
                        tunnel: [w398 w405] -> w384
                        tunnel: [w396 w404] -> w383
                        tunnel: w382 -> [_ _]
                        tunnel: w381 -> [w397 w403]
                        tunnel: w364 -> [w395 w402]
                        tunnel: [w395 w402] -> w363
                        frame False {
                          w396 = FALSE
                        }
                        frame True {
                          w404 = TRUE
                          n130 = Add(x=w403, y=1.0) -> (x+y=w408:dbl)
                          n131 = Add(x=w411, y="Delta T") -> (x+y=w410:dbl)
                        }
                      }
                      n132 = Wait (ms)(milliseconds to wait=u32 10) -> ()  [unwired: 1 out]
                      n133 = call <extravilib>:"Read.vi"("channel"=w368) -> ("element"=w367:bool)  [unwired: 1 in, 1 out]
                      n134 = Or(x=w366, y=w367) -> (x .or. y?=w365:bool)
                      "Increment" <- w382
                    }
                  }
                }
                "T0" <- w302
              }
            }
          }
          frame True {
            (unwired) 4.0
            # "n += 1"
            # "if(n == 1)"
            # "Initilaise T0 to first\ntemperature reading"
            n135 = Increment(x=w417) -> (x+1=w414:dbl)
            n136 = while {
              tunnel: w416 -> [w427]
              tunnel: [w420] -> w415
              stop <- w422 stop-if-true
              n137 = call <extravilib>:"Read.vi"("channel"=w427) -> ("element"=w426:waveform(dbl)[])  [unwired: 1 in, 1 out]
              "First read tag" <- w426
              n138 = Index Array(array=w426, index=0) -> (element=w425:waveform(dbl))
              n139 = Unbundle By Name(w425) -> ("Y"=w424:dbl[])
              n140 = call-poly <vilib>:"Mean.vi"("X"=w424) -> ("mean"=w421:dbl)  [unwired: 1 out]
              "mean" <- w421
              n141 = Not A Number/Path/Refnum?(number/path/refnum=w421) -> (NaN/Path/Refnum?=w423:bool)
              n142 = Not(x=w423) -> (.not. x?=w422:bool)
              n143 = case shown="False" w422 {
                tunnel: w421 -> [_ w430]
                tunnel: [1.0 ("mean") w430] -> w420
                frame False {
                }
                frame True {
                }
              }
            }
          }
        }
      }
      event User Event {
        n144 = event-data() -> ("element"=w447:T3)  [unwired: 1 in]
        n145 = Unbundle(w447) -> ("Command"=w446:string, "Data 2"=w438:variant, "Data 3"=w437:variant, "Data 4"=w434:variant)  [unwired: 1 out]
        n146 = case shown="\"DAQ Config\"" w446 {
          tunnel: w445 -> [w452 w457 w485 _ _ _ w521]
          tunnel: [w452 w457 w485 0 0 -1 w521] -> w444
          tunnel: w443 -> [w449 w454 w465 w492 w496 w506 w518]
          tunnel: [_ _ _ _ _ _ TRUE] -> w442
          tunnel: [w451 w456 w484 1.0 w498 w510 w519] -> w441
          tunnel: w440 -> [w451 w456 w484 _ w498 w510 w519]
          tunnel: w438 -> [_ _ w483 _ _ _ _]
          tunnel: w437 -> [_ _ w482 _ _ _ _]
          tunnel: w436 -> [w450 w455 w478 w490 w497 w503 w515]
          tunnel: [w450 w455 w477 w488 w497 w501 w514] -> w431
          tunnel: [w449 w454 w473 w491 w496 w504 w517] -> w435
          tunnel: w434 -> [_ _ w467 _ _ _ _]
          tunnel: [w448 w453 w463 w486 w495 w500 w512] -> w432
          tunnel: w433 -> [w448 w453 w463 w486 w495 w500 w512]
          frame Default {
          }
          frame "Choice Made" {
          }
          frame "DAQ Config" {
            w458 = 12573 items=["Active Drive"=12573, "Open Collector"=12574] ("DO.OutputDriveType")
            n147 = Variant To Data(error in=w465, type=tag "" ("Lines"), Variant=w483) -> (data=w469:tag, error out=w479:errorcluster)
            n148 = Variant To Data(error in=w465, type=refnum<visa-resource-name> refnum ("COM Port"), Variant=w482) -> (data=w476:refnum<visa-resource-name>, error out=w475:errorcluster)
            n149 = call-poly <vilib>:"DAQmx Create Virtual Channel.vi"("lines"=w469, "error in"=w479) -> ("task out"=w462:refnum<k21>, "error out"=w461:errorcluster)  [unwired: 12 in]
            n150 = call-poly "VISA Configure Serial Port"("VISA resource name"=w476, "Enable Termination\nChar (T)"=FALSE ("Enable Termination\nChar (T)"), "baud rate (9600)"=u32 115200, "error in (no error)"=w475) -> ("VISA resource name out"=w474:refnum<visa-resource-name>, "error out"=w472:errorcluster)  [unwired: 10 in]
            n151 = property class="DAQmx Channel"(reference=w462, error in=w461, "DO.OutputDriveType"=w458) -> (reference out=w459:refnum<k21>, error out=w460:errorcluster)
            n152 = Variant To Data(error in=w465, type=0.0, Variant=w467) -> (data=w466:dbl, error out=w464:errorcluster)
            n153 = Merge Errors(w464, w460, w472) -> (w473:errorcluster)
            n154 = Bundle By Name(cluster=w478, "Total Range"=w466, "Digital.DAQmx Task"=w459, "Serial.VISA name"=w474) -> (w477:T4)
          }
          frame "DAQ Start" {
            n155 = Unbundle By Name(w490) -> ("Digital.DAQmx Task"=w493:refnum<k21>)
            n156 = call <vilib>:"DAQmx Start Task.vi"("task/channels in"=w493, "error in"=w492) -> ("task out"=w489:refnum<k21>, "error out"=w491:errorcluster)  [unwired: 12 in]
            n157 = Bundle By Name(cluster=w490, "Digital.DAQmx Task"=w489) -> (w488:T4)
          }
          frame "Record" {
          }
          frame "DAQ Stop" {
            n158 = Unbundle By Name(w503) -> ("Digital.DAQmx Task"=w509:refnum<k21>)
            n159 = call <vilib>:"DAQmx Stop Task.vi"("task/channels in"=w509, "error in"=w506) -> ("task out"=w508:refnum<k21>, "error out"=w507:errorcluster)  [unwired: 12 in]
            n160 = Bundle By Name(cluster=w503, "Digital.DAQmx Task"=refnum<k21> refnum) -> (w501:T4)
            n161 = call <vilib>:"DAQmx Clear Task.vi"("task in"=w508, "error in"=w507) -> ("error out"=w505:errorcluster)  [unwired: 13 in]
            n162 = Merge Errors(w505) -> (w504:errorcluster)
          }
          frame "Exit" {
            n163 = Unbundle By Name(w515) -> ("Serial.VISA name"=w516:refnum<visa-resource-name>)
            n164 = VISA Close(VISA resource name=w516, error in (no error)=w518) -> (error out=w517:errorcluster)
            n165 = Bundle By Name(cluster=w515, "Serial.VISA name"=refnum<visa-resource-name> refnum) -> (w514:T4)
          }
        }
      }
    }
    n166 = call "Loop Error Stop.vi"("error in"=w207, "user event"=w218) -> ("error out"=w220:errorcluster)  [unwired: 9 in]
    "n" <- w215
  }
  n167 = Unregister For Events(event registration refnum=w12) -> ()  [unwired: 1 in, 1 out]
  n168 = call <extravilib>:"Replicate.vi"("stream"=w33) -> ("stream copy 1"=w7:T10, "stream copy 2"=w11:T10)  [unwired: 7 in]
  n169 = while {
    tunnel: w43 -> [w534]
    tunnel: [w533] -> w44
    tunnel: w11 -> [w531]
    shift-right: [w524] -> _
    shift-left: w20 -> [w530]
    shift-right: [w527] -> _
    shift-left: -1 -> [w528]
    shift-right: [w522] -> _
    shift-left: _ -> [w526]
    tunnel: w13 -> [w523]
    stop <- w532 stop-if-true
    # "File"
    n170 = call <extravilib>:"Read.vi"("channel"=w531) -> ("element"=w529:waveform(dbl)[])  [unwired: 6 in, 4 out]
    n171 = event shown="[1] <channel value>: User Event" {
      selector: w534 -> [_ _]
      dyn-events: [_ _] -> w533
      timeout: w528 -> [_ w557]
      tunnel: [w541 w563] -> w525
      tunnel: [_ w562] -> w532
      tunnel: w530 -> [w542 w558]
      tunnel: w529 -> [w540 _]
      tunnel: [w537 w556] -> w527
      tunnel: [w535 w555] -> w522
      tunnel: w526 -> [w539 _]
      event Timeout {
        n172 = event-data() -> ()  [unwired: 1 in, 1 out]
        n173 = case shown="False" w539 {
          tunnel: w542 -> [w546 w554]
          tunnel: [w546 w553] -> w541
          tunnel: w540 -> [w545 w551]
          tunnel: "Re Time" -> [_ w550]
          tunnel: [0 ("timeout") w549] -> w537
          tunnel: "Use Re Time" -> [_ w548]
          tunnel: [FALSE ("Recording") w547] -> w535
          frame False {
            # "Read element out"
            "element" <- w545
          }
          frame True {
            # "Save element"
            n174 = call "File Manager.vi"("Use Record Time"=w548, "Record Time (s)"=w550, "Enum"=File_Manager_Enum."Volt Data", "error in"=w554, "Voltage"=w551) -> ("error out"=w553:errorcluster, "Recording"=w547:bool, "timeout"=w549:i32)  [unwired: 3 in, 1 out]
          }
        }
      }
      event User Event {
        n175 = event-data() -> ("element"=w561:T3)  [unwired: 1 in]
        n176 = Unbundle(w561) -> ("Command"=w560:string, "Data"=w559:variant)  [unwired: 3 out]
        n177 = case shown="\"Exit\"" w560 {
          tunnel: [w564 w570 w579 w582 w584 w586 w591] -> w563
          tunnel: [_ _ _ _ _ _ TRUE] -> w562
          tunnel: w559 -> [_ _ w578 _ _ _ _]
          tunnel: w558 -> [w564 w566 w574 w582 w584 w587 w591]
          tunnel: w557 -> [w565 w567 w573 _ _ _ w593]
          tunnel: [w565 w567 w573 0 0 -1 w593] -> w556
          tunnel: [_ _ _ _ TRUE FALSE _] -> w555
          frame Default {
          }
          frame "Choice Made" {
            n178 = call "File Manager.vi"("Enum"=File_Manager_Enum."Create File", "error in"=w566, "File Choice"="File Choice", "File Name"="File Name") -> ("error out"=w570:errorcluster, "File Path"=→"File Path":path)  [unwired: 4 in, 2 out]
          }
          frame "DAQ Config" {
            n179 = Variant To Data(error in=w574, type=T9 {"Index"=[], "Chl Name"=[], "Scale"=[], "Offset"=[], "Sample Rate"=100, "Device Name"="", "Channel"=""} ("Volt Channel"), Variant=w578) -> (data=w575:T9, error out=w576:errorcluster)
            n180 = call "File Manager.vi"("Volt Channel"=w575, "Enum"=File_Manager_Enum."Config Data", "error in"=w576) -> ("error out"=w579:errorcluster)  [unwired: 5 in, 3 out]
          }
          frame "DAQ Start" {
          }
          frame "Record" {
          }
          frame "DAQ Stop" {
            n181 = call "File Manager.vi"("Enum"=File_Manager_Enum."Close File", "error in"=w587) -> ("error out"=w586:errorcluster)  [unwired: 6 in, 3 out]
          }
          frame "Exit" {
          }
        }
      }
    }
    "Recording" <- w522
    n182 = call "Loop Error Stop.vi"("error in"=w525, "user event"=w523) -> ("error out"=w524:errorcluster)  [unwired: 9 in]
  }
  n183 = while {
    tunnel: w41 -> [w604]
    tunnel: [w603] -> w40
    shift-right: [w600] -> _
    shift-left: -1 -> [w601]
    tunnel: w7 -> [w599]
    shift-right: [w595] -> _
    shift-left: _ -> [w597]
    tunnel: w13 -> [w594]
    stop <- w602 stop-if-true
    # "Data Display"
    n184 = call <extravilib>:"Read.vi"("channel"=w599) -> ("element"=w598:waveform(dbl)[])  [unwired: 6 in, 4 out]
    n185 = event shown="[1] <channel value>: User Event" {
      selector: w604 -> [_ _]
      dyn-events: [_ _] -> w603
      timeout: w601 -> [w607 w615]
      tunnel: [_ w620] -> w602
      tunnel: [w611 w619] -> w596
      tunnel: [w607 w614] -> w600
      tunnel: w598 -> [w609 w612]
      tunnel: w597 -> [w608 w613]
      event Timeout {
        n186 = event-data() -> ()  [unwired: 1 in, 1 out]
        n187 = call "Data Display Manager.vi"("Enum"=Data_Display_Manager_Enum."Volt Data", "error in"=w608, "Raw Data"=w609) -> ("error out"=w611:errorcluster, "Overall Mean"=→"Overall Raw \nVoltage Mean":dbl[], "Mean per Second"=→"Raw Voltage Mean \nper Second":dbl[])  [unwired: 5 in, 1 out]
      }
      event User Event {
        n188 = event-data() -> ("element"=w618:T3)  [unwired: 1 in]
        n189 = Unbundle(w618) -> ("Command"=w617:string, "Data"=w616:variant)  [unwired: 3 out]
        n190 = case shown="\"Exit\"" w617 {
          tunnel: [_ _ _ _ _ _ TRUE] -> w620
          tunnel: [w621 w625 w636 w639 w641 w646 w648] -> w619
          tunnel: w616 -> [_ _ w634 _ _ _ _]
          tunnel: w615 -> [w622 w624 w638 _ _ _ w649]
          tunnel: [w622 w624 w638 0 0 -1 w649] -> w614
          tunnel: w613 -> [w621 w623 w631 w639 w642 w646 w648]
          tunnel: w612 -> [_ _ _ _ w643 _ _]
          frame Default {
          }
          frame "Choice Made" {
            n191 = control-ref of="DD SubPane"() -> (w628:refnum<vi>)
            n192 = call "Data Display Manager.vi"("Enum"=Data_Display_Manager_Enum."Display Choice", "error in"=w623, "Data Display Choice"="DD Choice") -> ("error out"=w626:errorcluster, "VI Ref"=w627:refnum<vi>)  [unwired: 5 in, 2 out]
            n193 = call "Insert Panel to Subpanel.vi"("SubPanel in"=w628, "error in"=w626, "VI Ref"=w627) -> ("error out"=w625:errorcluster)  [unwired: 8 in]
          }
          frame "DAQ Config" {
            n194 = Variant To Data(error in=w631, type=T9 {"Index"=[], "Chl Name"=[], "Scale"=[], "Offset"=[], "Sample Rate"=100, "Device Name"="", "Channel"=""} ("Volt Channel"), Variant=w634) -> (data=w632:T9, error out=w633:errorcluster)
            n195 = call "Data Display Manager.vi"("Volt Channel"=w632, "Enum"=Data_Display_Manager_Enum."Config Data", "error in"=w633) -> ("error out"=w636:errorcluster)  [unwired: 5 in, 3 out]
          }
          frame "DAQ Start" {
          }
          frame "Record" {
            # "continuous displaying when user\npressed Record."
            n196 = call "Data Display Manager.vi"("Enum"=Data_Display_Manager_Enum."Volt Data", "error in"=w642, "Raw Data"=w643) -> ("error out"=w641:errorcluster)  [unwired: 5 in, 3 out]
          }
          frame "DAQ Stop" {
          }
          frame "Exit" {
          }
        }
      }
    }
    n197 = call "Loop Error Stop.vi"("error in"=w596, "user event"=w594) -> ("error out"=w595:errorcluster)  [unwired: 9 in]
  }
  n198 = Unregister For Events(event registration refnum=w39) -> ()  [unwired: 1 in, 1 out]
  n199 = Unregister For Events(event registration refnum=w40) -> ()  [unwired: 1 in, 1 out]
  n200 = Unregister For Events(event registration refnum=w44) -> ()  [unwired: 1 in, 1 out]
